vi "Actor Core original.vi"(8 "error in":errorcluster, 11 "Waveform Plot in":refnum<class "Waveform Plot.lvclass">) -> (0 "error out":errorcluster, 3 "Actor out":refnum<class "Actor.lvclass">)   [LabVIEW 2015]
doc: "(<B>Filename</B>: Actor Framework.lvlib:Actor.lvclass:Actor Core.vi)\n\nReceives messages to the actor, reacts to them, and initiates any error handling that may shut the actor down.\n\nDescendant classes may override this VI to append parallel tasks for the actor to complete while it handles messages. Overrides use the Call Parent Method node."
uses:
  Waveform Plot.lvclass
  <vilib>/ActorFramework/Actor/Actor.lvclass
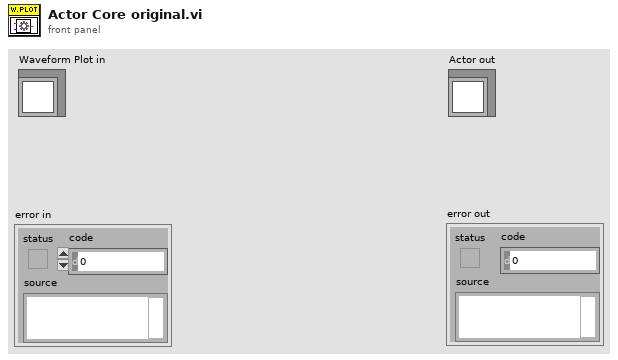
[diagram p1: front panel]
types:
  T1 = cluster{"File Path Control":path, "Group":string, "Channel":string, "Abbreviated":string}[]
  T2 = cluster{"File Path Control":path, "Group":string, "Channel":string, "Abbreviated":string}
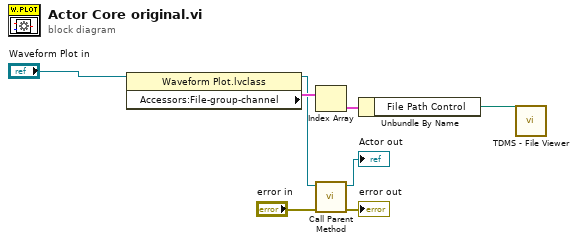
[diagram p0: block diagram]
diagram:
  n1 = property class="Waveform Plot.lvclass"(reference="Waveform Plot in") -> (reference out=w2:refnum<class "Waveform Plot.lvclass">, "Accessors:File-group-channel"=w5:T1)  [unwired: 1 in, 1 out]
  n2 = Index Array(array=w5) -> (element=w4:T2)  [unwired: 1 in]
  n3 = call-parent "Call Parent Method"("error in"="error in", "Measure Object in"=w2) -> ("error out"=→"error out":errorcluster, "Actor out"=→"Actor out":refnum<class "Actor.lvclass">)  [unwired: 8 in]
  n4 = Unbundle By Name(w4) -> ("File Path Control"=w1:path)
  n5 = call <vilib>:"TDMS - File Viewer.vi"("file path"=w1) -> ()  [unwired: 5 in, 2 out]
